vi "Get SMO Serial Number.vi"(8 "error in (no error)":errorcluster, 11 "Inst.Krohn-Hite-7008 in":refnum<class "Inst.Krohn-Hite-7008.lvclass">) -> (0 "error out":errorcluster, 2 "Serial Number":string, 3 "Inst.Krohn-Hite-7008 out":refnum<class "Inst.Krohn-Hite-7008.lvclass">)   [LabVIEW 2019, in "Inst.Krohn-Hite-7008.lvclass"]
doc: "Override this VI to return the serial number of your Instrument"
uses:
  Inst.Krohn-Hite-7008.lvclass
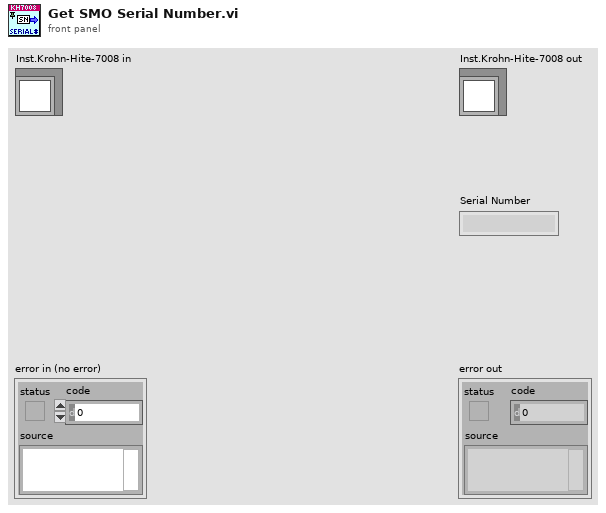
[diagram p1: front panel]
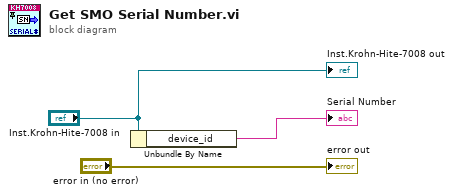
[diagram p0: block diagram]
diagram:
  n1 = Unbundle By Name("Inst.Krohn-Hite-7008 in") -> ("device_id"=→"Serial Number":string)
  "error out" <- "error in (no error)"
  "Inst.Krohn-Hite-7008 out" <- "Inst.Krohn-Hite-7008 in"
